vi "Lab_4_1.vi"() -> ()   [LabVIEW 2018]
panel:
  in  "milliseconds to wait":u32
  out "Waveform Graph":i32[](graph)
  out "Final value":dbl
  out "The iteration":dbl
  in  "Numeric":i32
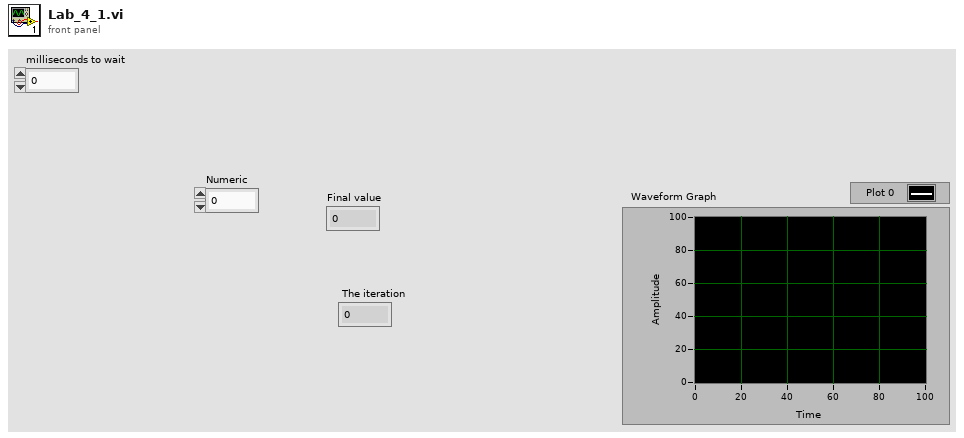
[diagram p1: front panel]
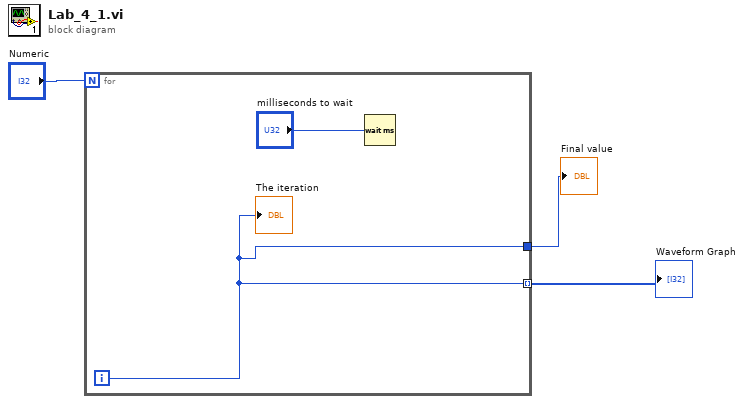
[diagram p0: block diagram]
diagram:
  n1 = for {
    N: "Numeric" -> [_]
    tunnel: [w5] -> w2
    tunnel: [w5] -> w1 mode=indexing
    i -> [w5]
    n2 = Wait (ms)(milliseconds to wait="milliseconds to wait") -> ()  [unwired: 1 out]
    "The iteration" <- w5
  }
  "Final value" <- w2
  "Waveform Graph" <- w1
